vi "FileOperationWrite.vi"() -> ()   [LabVIEW 2019]
panel:
  in  "?":path
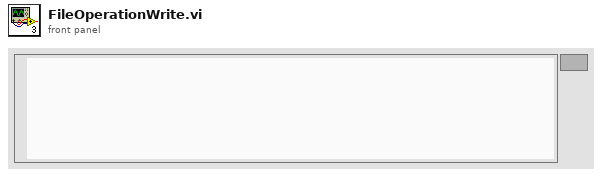
[diagram p1: front panel]
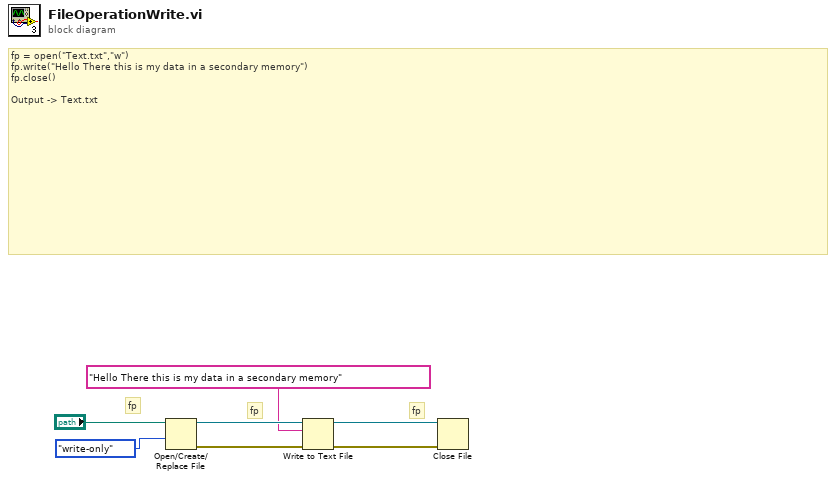
[diagram p0: block diagram]
diagram:
  # "fp"
  # "fp"
  # "fp"
  # "fp = open(\"Text.txt\",\"w\")\nfp.write(\"Hello There this is my data in a secondary memory\")\nfp.close()\n\nOutput -> Text.txt"
  n1 = Open/Create/Replace File(file path (use dialog)="?", access (0:read/write)=enum16{"read/write", "read-only", "write-only"}."write-only") -> (refnum out=w5:refnum<file>, error out=w4:errorcluster)  [unwired: 4 in, 1 out]
  n2 = Write to Text File(file (use dialog)=w5, text="Hello There this is my data in a secondary memory", error in=w4) -> (refnum out=w2:refnum<file>, error out=w3:errorcluster)  [unwired: 1 in, 1 out]
  n3 = Close File(refnum=w2, error in=w3) -> ()  [unwired: 2 out]
